vi "objectiffunctionmatlab.vi"(8 "error in (no error)":errorcluster, 11 "Table Control":string[][](array[string])) -> (0 "error out":errorcluster, 3 "objective function":string)   [LabVIEW 2019]
panel:
  out "concatenated string":string
  out "données plantes":string
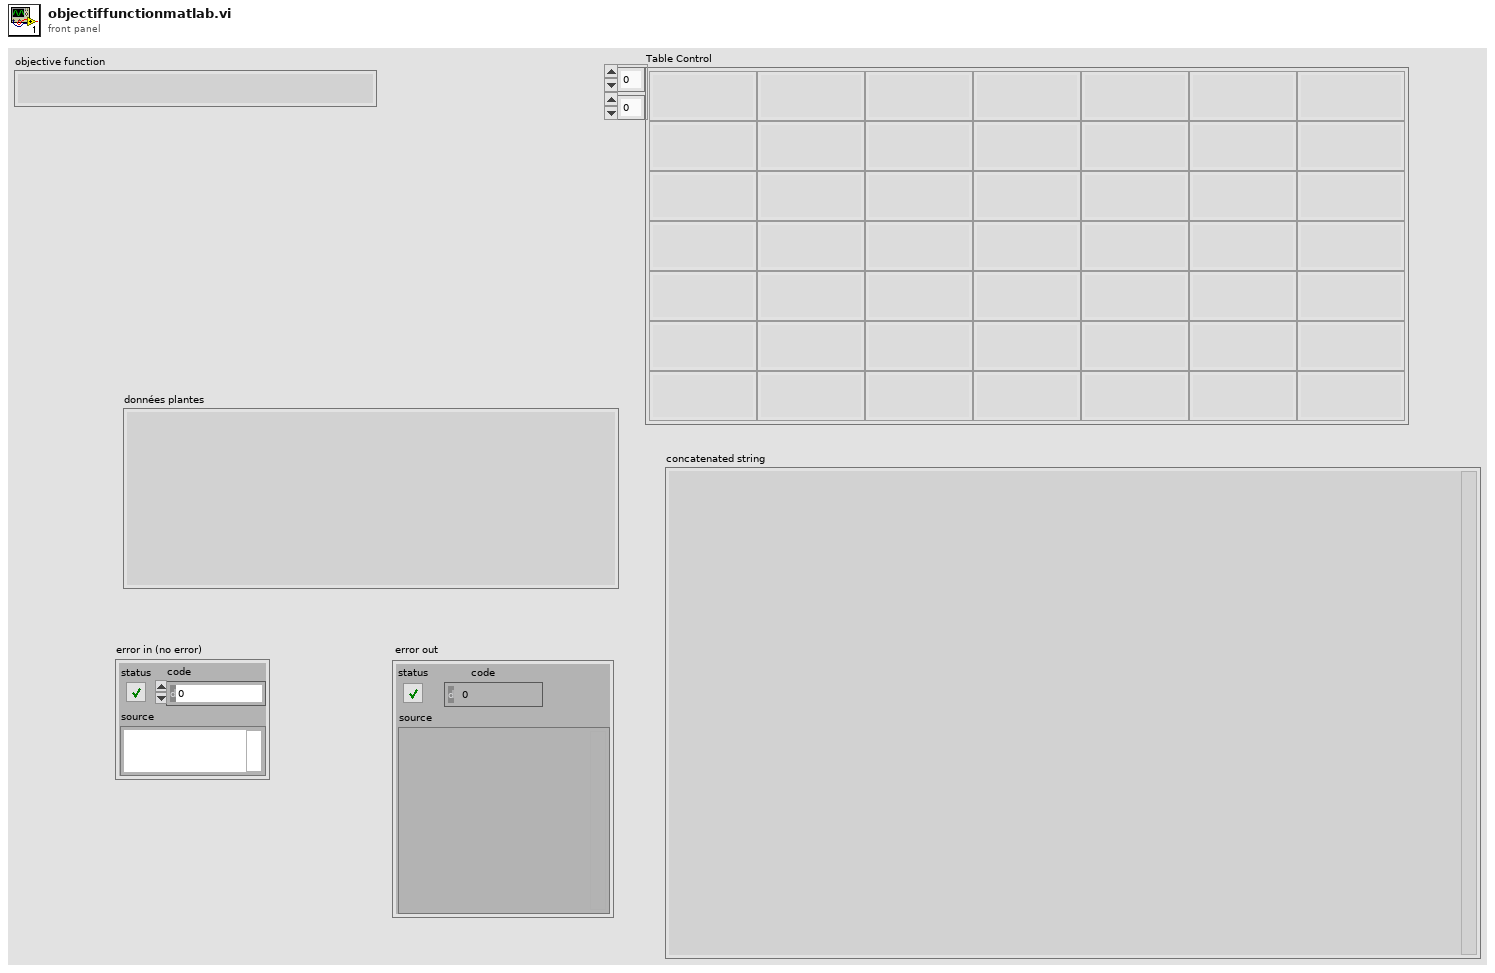
[diagram p1: front panel]
types:
  T1 = enum16{"open", "replace", "create", "open or create", "replace or create", "replace or create with confirmation"}
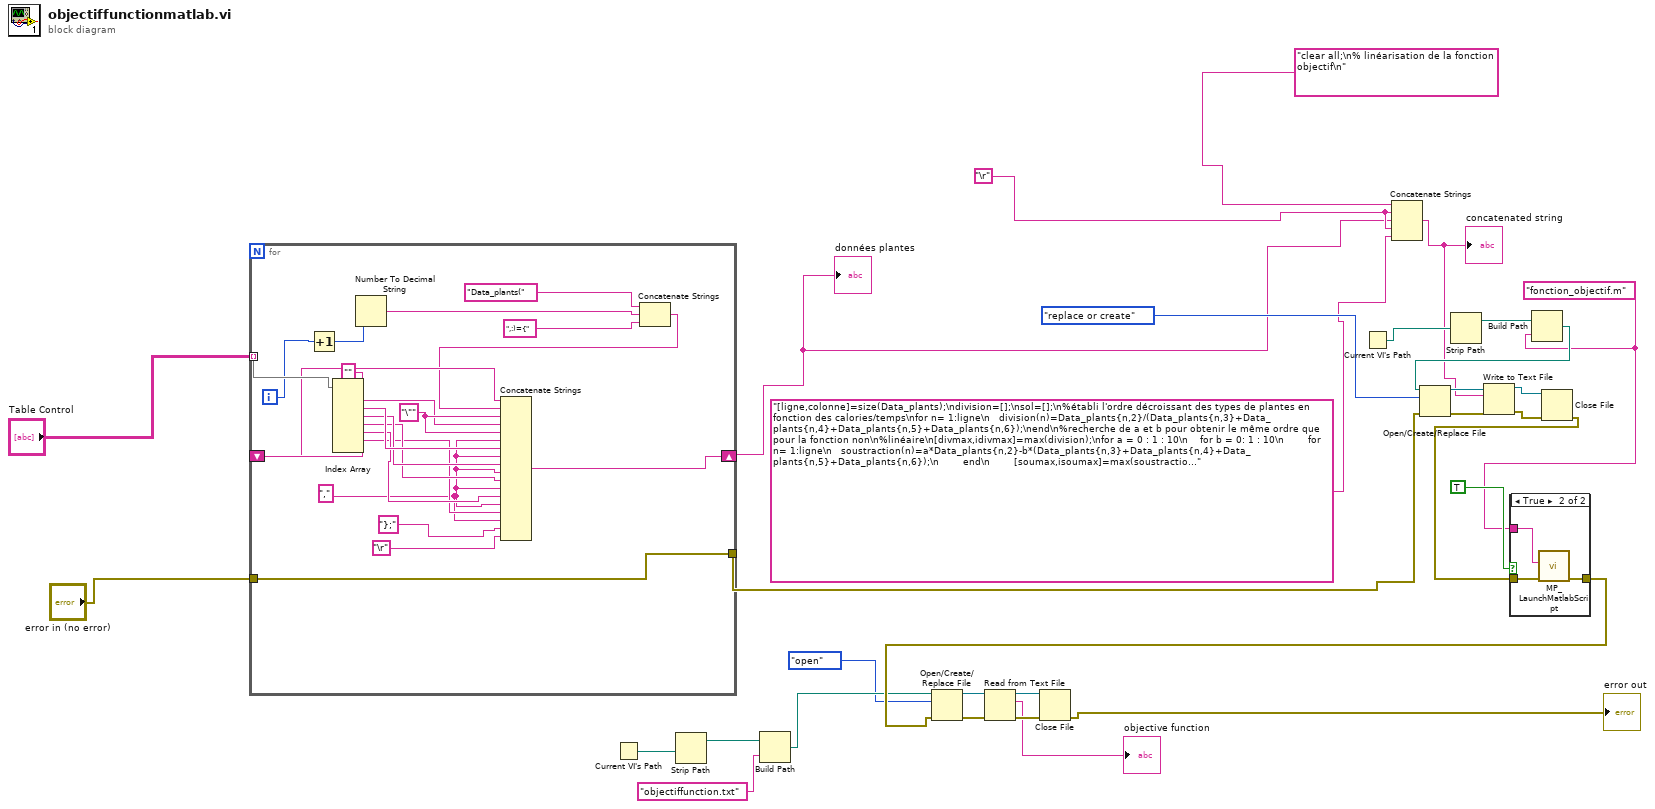
[diagram p0: block diagram]
diagram:
  w16 = "fonction_objectif.m"
  w14 = "\r"
  n1 = for {
    tunnel: "Table Control" -> [w52] mode=indexing
    shift-right: [w51] -> w13
    shift-left: "" -> [w50]
    tunnel: "error in (no error)" -> [w33]
    tunnel: [w33] -> w20
    i -> [w49]
    w43 = "\""
    w36 = ","
    n2 = Increment(x=w49) -> (x+1=w48:i32)
    n3 = Index Array(array=w52) -> (element #1=w42:string, element #2=w41:string, element #3=w40:string, element #4=w39:string, element #5=w38:string, element #6=w37:string)  [unwired: 7 in, 1 out]
    n4 = Number To Decimal String(number=w48) -> (decimal integer string=w47:string)  [unwired: 1 in]
    n5 = Concatenate Strings("Data_plants(", w47, ",:)={") -> (w44:string)
    n6 = Concatenate Strings(w50, w44, w43, w42, w43, w36, w41, w36, w40, w36, w39, w36, w38, w36, w37, w36, "};", "\r") -> (w51:string)
  }
  "données plantes" <- w13
  n7 = Current VI's Path() -> (path=w6:path)
  n8 = Strip Path(path=w6) -> (stripped path=w4:path)  [unwired: 1 out]
  n9 = Build Path(base path=w4, name or relative path="objectiffunction.txt") -> (appended path=w5:path)
  n10 = Current VI's Path() -> (path=w25:path)
  n11 = Concatenate Strings("clear all;\n% linéarisation de la fonction objectif\n", w14, w13, w14, "[ligne,colonne]=size(Data_plants);\ndivision=[];\nsol=[];\n%établi l'ordre décroissant des types de plantes en fonction des calories/temps\nfor n= 1:ligne\n   division(n)=Data_plants{n,2}/(Data_plants{n,3}+Data_plants{n,4}+Data_plants{n,5}+Data_plants{n,6});\nend\n%recherche de a et b pour obtenir le même ordre que pour la fonction non\n%linéaire\n[divmax,idivmax]=max(division);\nfor a = 0 : 1 : 10\n    for b = 0: 1 : 10\n        for n= 1:ligne\n   soustraction(n)=a*Data_plants{n,2}-b*(Data_plants{n,3}+Data_plants{n,4}+Data_plants{n,5}+Data_plants{n,6});\n        end\n        [soumax,isoumax]=max(soustraction);\n        if (isoumax==idivmax)\n           sol=[sol,a,b]; \n        end\n    end\nend\n\nfid = fopen('objectiffunction.txt','wt');\nfprintf(fid, 'm.Maximize(%d * total_calories - %d * total_growtime)', sol(end-1), sol(end));\nfclose(fid);") -> (w21:string)
  "concatenated string" <- w21
  n12 = Strip Path(path=w25) -> (stripped path=w24:path)  [unwired: 1 out]
  n13 = Build Path(base path=w24, name or relative path=w16) -> (appended path=w23:path)
  n14 = Open/Create/Replace File(file path (use dialog)=w23, error in=w20, operation (0:open)=T1."replace or create") -> (refnum out=w27:refnum<file>, error out=w19:errorcluster)  [unwired: 3 in, 1 out]
  n15 = Write to Text File(file (use dialog)=w27, text=w21, error in=w19) -> (refnum out=w26:refnum<file>, error out=w18:errorcluster)  [unwired: 1 in, 1 out]
  n16 = Close File(refnum=w26, error in=w18) -> (error out=w17:errorcluster)  [unwired: 1 out]
  n17 = case shown="True" TRUE {
    tunnel: w17 -> [w53 w56]
    tunnel: [w53 w55] -> w10
    tunnel: w16 -> [_ w54]
    frame False {
    }
    frame True {
      n18 = call "MP_LaunchMatlabScript.vi"("error in (no error)"=w56, "matlab script name with extension"=w54) -> ("error out"=w55:errorcluster)  [unwired: 5 in, 4 out]
    }
  }
  n19 = Open/Create/Replace File(file path (use dialog)=w5, error in=w10, operation (0:open)=T1."open") -> (refnum out=w11:refnum<file>, error out=w12:errorcluster)  [unwired: 3 in, 1 out]
  n20 = Read from Text File(file (use dialog)=w11, error in=w12) -> (refnum out=w8:refnum<file>, text=→"objective function":string, error out=w9:errorcluster)  [unwired: 2 in, 1 out]
  n21 = Close File(refnum=w8, error in=w9) -> (error out=→"error out":errorcluster)  [unwired: 1 out]
